vi "Create Transfer Group Configuration.vi"(8 "error in (no error)":errorcluster, 10 "Transfer Group Configuration":T1, 11 "Transfer Group Configuration in":refnum<class "Transfer Group Configuration.lvclass">) -> (0 "error out":errorcluster, 3 "Transfer Group Configuration out":refnum<class "Transfer Group Configuration.lvclass">)   [LabVIEW 2017, in "DSF Core.lvlib" / "Transfer Group Configuration.lvclass"]
uses:
  Transfer Group Configuration.lvclass
  DSF Configuration API/Public/Controls/DSF Engine Transfer Group Configuration.ctl
  DSF Configuration API/Public/Controls/DSF Direction.ctl
  DSF Configuration API/Public/Controls/DSF Timing Info.ctl
  DSF Configuration API/Public/Controls/DSF Engine Transfer Configuration.ctl
  DSF Configuration API/Public/Controls/DSF Byte Order.ctl
  DSF Configuration API/Public/Controls/DSF Engine Channel Configuration.ctl
  DSF Configuration API/Public/Controls/DSF Data Type.ctl
  DSF Configuration API/Public/Controls/DSF Settings Info.ctl
  Transfer/Transfer Configuration.lvclass
  Transfer Group Configuration.lvclass/Transfer Group Configuration.ctl
  DSF Core.lvlib
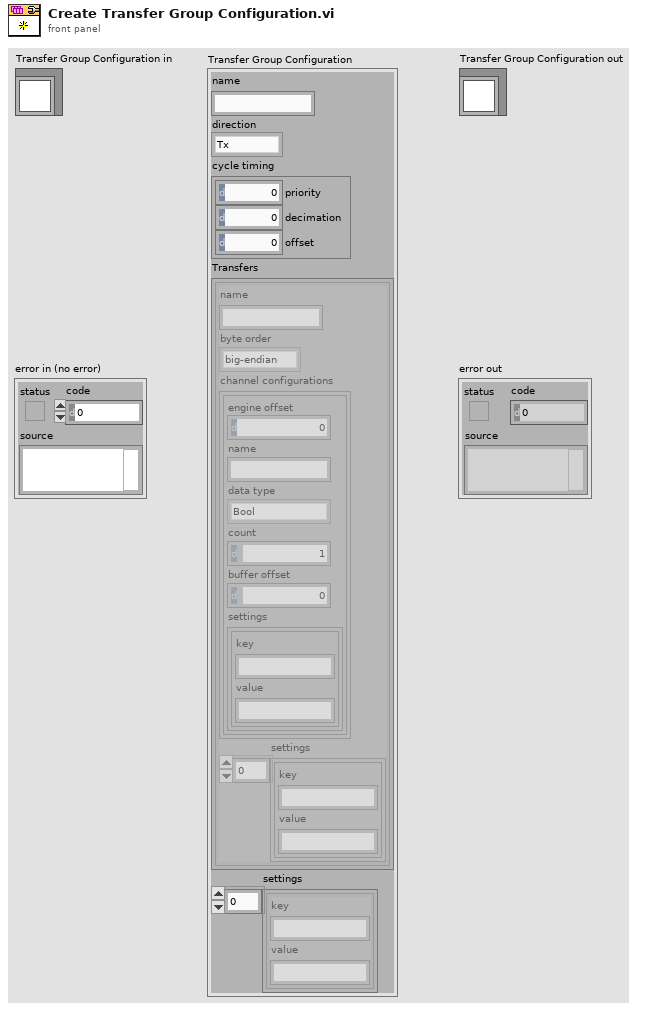
[diagram p1: front panel]
types:
  T1 = typedef "DSF Core.lvlib/DSF Engine Transfer Group Configuration.ctl" = cluster{"name":string, "direction":T2, "cycle timing":T3, "Transfers":T4[], "settings":T8}
  T2 = typedef "DSF Core.lvlib/DSF Direction.ctl" = enum8{"Tx", "Rx"}
  T3 = typedef "DSF Core.lvlib/DSF Timing Info.ctl" = cluster{"priority":u64, "decimation":u64, "offset":u64}
  T4 = typedef "DSF Core.lvlib/DSF Engine Transfer Configuration.ctl" = cluster{"name":string, "byte order":T5, "channel configurations":T6[], "settings":T8}
  T5 = typedef "DSF Core.lvlib/DSF Byte Order.ctl" = enum8{"big-endian", "little-endian"}
  T6 = typedef "DSF Core.lvlib/DSF Engine Channel Configuration.ctl" = cluster{"engine offset":u64, "name":string, "data type":T7, "count":u64, "buffer offset":u64, "settings":T8}
  T7 = typedef "DSF Core.lvlib/DSF Data Type.ctl" = enum8{"Bool", "SGL", "DBL", "I8", "I16", "I32", "I64", "U8", "U16", "U32", "U64"}
  T8 = typedef "DSF Core.lvlib/DSF Settings Info.ctl" = cluster{"key":string, "value":string}[]
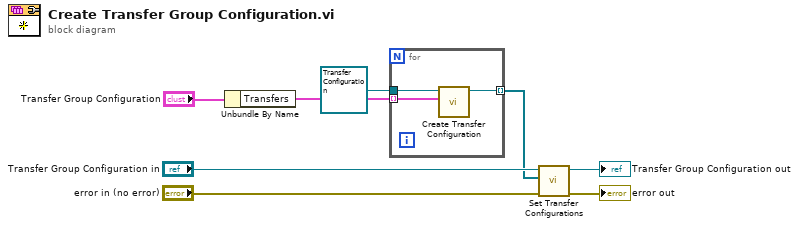
[diagram p0: block diagram]
diagram:
  n1 = Unbundle By Name("Transfer Group Configuration") -> ("Transfers"=w5:T4[])
  n2 = for {
    tunnel: w5 -> [w10] mode=indexing
    tunnel: refnum<class "Transfer Configuration.lvclass"> refnum ("Transfer Configuration in") -> [w9]
    tunnel: [w8] -> w1 mode=indexing
    n3 = call "Create Transfer Configuration.vi"("Transfer Configuration"=w10, "Transfer Configuration in"=w9) -> ("Transfer Configuration out"=w8:refnum<class "Transfer Configuration.lvclass">)  [unwired: 8 in, 1 out]
  }
  n4 = call "Set Transfer Configurations.vi"("Transfer Configurations"=w1, "Transfer Group Configuration in"="Transfer Group Configuration in") -> ("Transfer Group Configuration out"=→"Transfer Group Configuration out":refnum<class "Transfer Group Configuration.lvclass">)  [unwired: 9 in]
  "error out" <- "error in (no error)"
